vi "Export Custom SCP Commands List.vi"(8 "error in (no error)":errorcluster, 11 "Node Ptr":u64 format="%.0x") -> (0 "error out":errorcluster)   [LabVIEW 2018, in "Vires VTD System Explorer.lvlib"]
uses:
  Vires VTD System Explorer.lvlib
  <vilib>/Utility/file.llb/Write Delimited Spreadsheet (string).vi
  <vilib>/NI Veristand/Custom Device Tools/Custom Device Utility Library/Custom Device Utility Library.lvlib
panel:
  in  "Tag":string
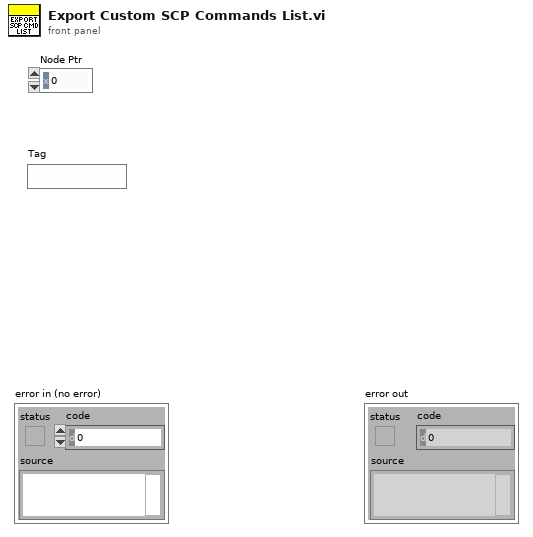
[diagram p1: front panel]
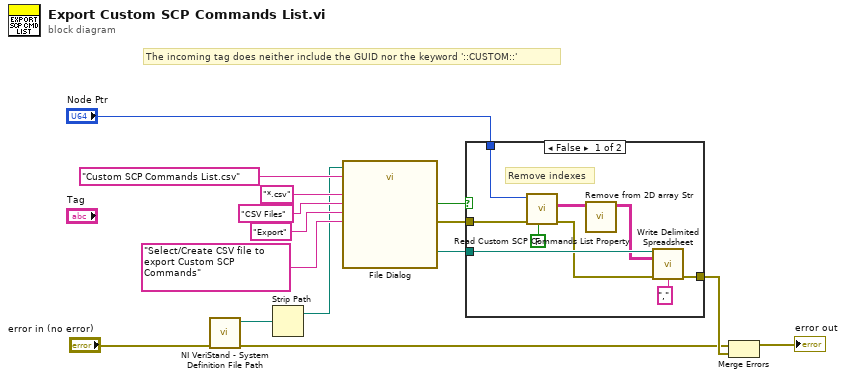
[diagram p0: block diagram]
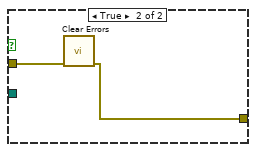
[diagram p2: hidden frame]
diagram:
  # "The incoming tag does neither include the GUID nor the keyword '::CUSTOM::'"
  n1 = call <vilib>:"NI VeriStand - System Definition File Path.vi"("error in (no error)"="error in (no error)") -> ("error out"=w2:errorcluster, "SDF path"=w4:path)  [unwired: 9 in]
  n2 = Strip Path(path=w4) -> (stripped path=w1:path)  [unwired: 1 out]
  n3 = call "File Dialog"("start path"=w1, "prompt"="Select/Create CSV file to export Custom SCP Commands", "button label"="Export", "default name"="Custom SCP Commands List.csv", "pattern (all files)"="*.csv", "pattern label"="CSV Files") -> ("selected path"=w9:path, "cancelled"=w10:bool, "error out"=w8:errorcluster)  [unwired: 6 in, 1 out]
  n4 = case shown="False" w10 {
    tunnel: w9 -> [w24 _]
    tunnel: w8 -> [w21 w26]
    tunnel: [w23 w25] -> w7
    tunnel: "Node Ptr" -> [w22 _]
    frame False {
      # "Remove indexes"
      n5 = call "Read Custom SCP Commands List Property.vi"("Add 1st Column Idx? (T)"=FALSE, "error in (no error)"=w21, "Node Ptr"=w22) -> ("error out"=w20:errorcluster, "Custom SCP Commands List"=w19:string[][])  [unwired: 6 in, 1 out]
      n6 = call "Remove from 2D array Str.vi"("Strings In"=w19) -> ("Result Strings Out"=w16:string[][])  [unwired: 10 in]
      n7 = call-poly <vilib>:"Write Delimited Spreadsheet.vi"("file path (dialog if empty)"=w24, "2D data"=w16, "error in (no error)"=w20, "delimiter (\\t)"="," ("delimiter (\\t)")) -> ("error out"=w23:errorcluster)  [unwired: 10 in, 1 out]
    }
    frame True {
      n8 = call <vilib>:"Clear Errors.vi"("error in (no error)"=w26) -> ("error out"=w25:errorcluster)  [unwired: 5 in, 1 out]
    }
  }
  n9 = Merge Errors(w2, w7) -> (→"error out":errorcluster)
